vi "JLINKARM Read Mem U32.vi"(7 "flag":u32, 8 "error in (no error)":errorcluster caption="错误输入（无错误）", 9 "buff":u32, 10 "size":u32, 11 "memaddr":u32) -> (0 "error out":errorcluster caption="错误输出", 1 "buff out":u32, 3 "function return":i32)   [LabVIEW 2016, in "JLinkARM.lvlib"]
doc: "int JLINKARM_ReadMemU32(unsigned long memaddr,unsigned long size,unsigned long * buff,unsigned long flag);"
uses:
  <userlib>/LV-JLinkARM/JLinkARM.lvlib
  <userlib>/LV-JLinkARM/JLinkARM.dll
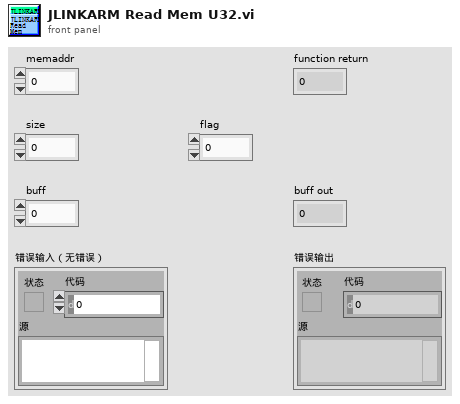
[diagram p1: front panel]
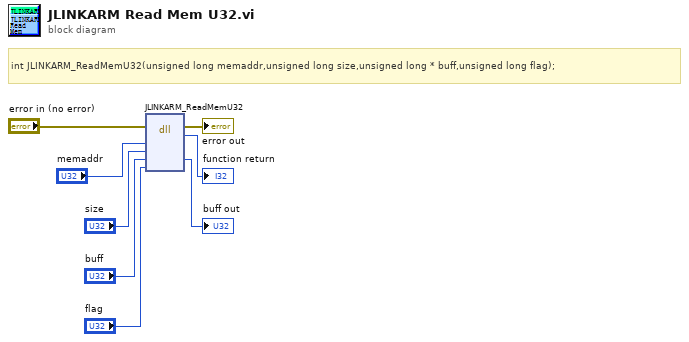
[diagram p0: block diagram]
diagram:
  # "int JLINKARM_ReadMemU32(unsigned long memaddr,unsigned long size,unsigned long * buff,unsigned long flag);"
  n1 = dll-call lib="C:/Program Files (x86)/National Instruments/LabVIEW 2016/user.lib/LV-JLinkARM/JLinkARM.*" fn="JLINKARM_ReadMemU32"(error in="error in (no error)", "memaddr"="memaddr", "size"="size", "buff"="buff", "flag"="flag") -> (error out=→"error out":errorcluster, →"function return":i32, "buff"=→"buff out":u32)  [unwired: 5 in, 1 out]
